vi "CreateListener.vi"(8 "error in (no error)":errorcluster, 9 "remote port":u16=54165, 11 "TCPIP in":refnum<class "TCPIP.lvclass">) -> (0 "error out":errorcluster, 3 "TCPIP out":refnum<class "TCPIP.lvclass">)   [LabVIEW 2018, in "TCPIP.lvclass"]
uses:
  TCPIP.lvclass
  TCPIP.lvclass/TCPIP.ctl
panel:
  out "port":u16
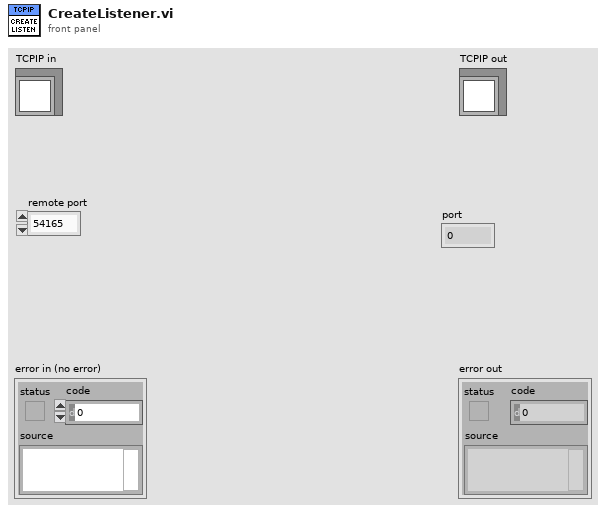
[diagram p1: front panel]
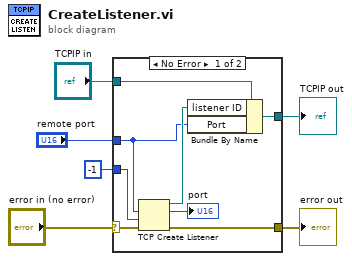
[diagram p0: block diagram]
diagram:
  n1 = case shown="No Error" "error in (no error)" {
    selector: "error in (no error)" -> [w9 w16]
    tunnel: [w8 w16] -> w5
    tunnel: [w13 w15] -> w3
    tunnel: "TCPIP in" -> [w14 w15]
    tunnel: "remote port" -> [w11 _]
    tunnel: -1 ("timeout") -> [w10 _]
    frame No Error {
      n2 = TCP Create Listener(8:w9, 9:w10, 10:w11) -> (0:w8:errorcluster, 2:→"port":u16, 3:w12:refnum<k5>)  [unwired: 2 in]
      n3 = Bundle By Name(cluster=w14, "listener ID"=w12, "Port"=w11) -> (w13:refnum<class "TCPIP.lvclass">)
    }
    frame Error {
    }
  }
  "error out" <- w5
  "TCPIP out" <- w3
